vi "Eas_encryption.vi"(8 "error in":errorcluster, 10 "Key":string, 11 "User":string) -> (0 "Error out":errorcluster, 2 "Key":string, 3 "User":string)   [LabVIEW 2016]
uses:
  <vilib>/Alab Technologies/AES Crypto/Controls/Key Length.ctl
  <vilib>/Alab Technologies/AES Crypto/AES Crypto.lvlib
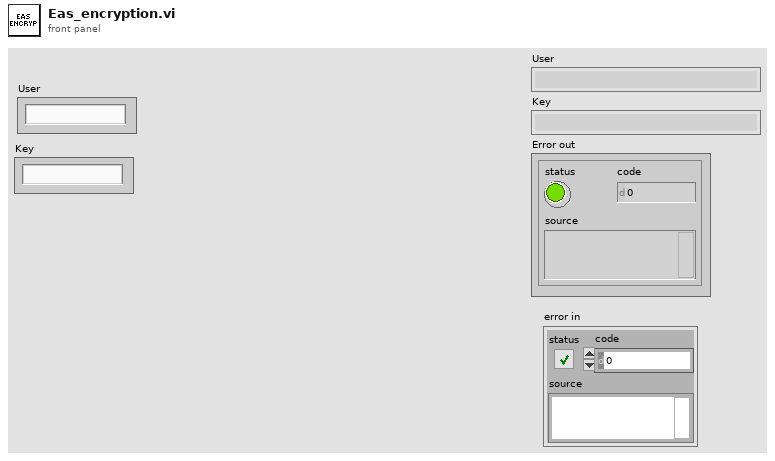
[diagram p1: front panel]
types:
  T1 = typedef "AES Crypto.lvlib/Key Length.ctl" = enum16{"128", "192", "256"}
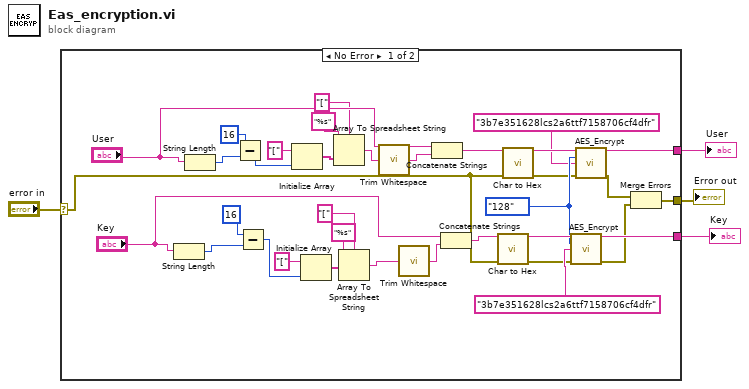
[diagram p0: block diagram]
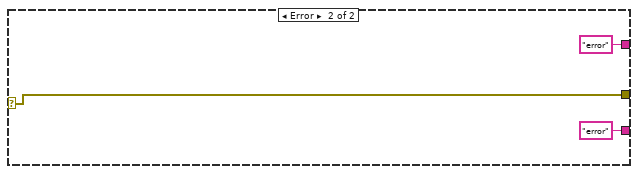
[diagram p2: hidden frame]
diagram:
  n1 = case shown="No Error" "error in" {
    selector: "error in" -> [w10 w42]
    tunnel: [w12 "error" ("Ciphertext (hex)")] -> w4
    tunnel: [w11 "error" ("Ciphertext (hex)")] -> w3
    tunnel: [w5 w42] -> w1
    frame No Error {
      w15 = Key_Length."128" ("Key length")
      n2 = String Length(string="Key") -> (length=w22:i32)
      n3 = String Length(string="User") -> (length=w24:i32)
      n4 = Subtract(x=16 ("y"), y=w24) -> (x-y=w36:i32)
      n5 = Subtract(x=16 ("y"), y=w22) -> (x-y=w38:i32)
      n6 = Initialize Array("[", w36) -> (w35:string[])
      n7 = Initialize Array("[", w38) -> (w34:string[])
      n8 = Array To Spreadsheet String(delimiter (Tab)="[", array=w35, 3:"%s" ("format string")) -> (spreadsheet string=w27:string)
      n9 = Array To Spreadsheet String(delimiter (Tab)="[", array=w34, 3:"%s" ("format string")) -> (spreadsheet string=w29:string)
      n10 = call <vilib>:"Trim Whitespace.vi"("string"=w27) -> ("trimmed string"=w26:string)  [unwired: 1 in]
      n11 = call <vilib>:"Trim Whitespace.vi"("string"=w29) -> ("trimmed string"=w28:string)  [unwired: 1 in]
      n12 = Concatenate Strings("User", w26) -> (w19:string)
      n13 = Concatenate Strings("Key", w28) -> (w17:string)
      n14 = call <vilib>:"Char to Hex.vi"("Input string (char)"=w17, "error in (no error)"=w10) -> ("Output string (hex)"=w16:string, "error out"=w9:errorcluster)  [unwired: 12 in]
      n15 = call <vilib>:"Char to Hex.vi"("Input string (char)"=w19, "error in (no error)"=w10) -> ("Output string (hex)"=w18:string, "error out"=w8:errorcluster)  [unwired: 12 in]
      n16 = call <vilib>:"AES_Encrypt.vi"("Plain text (hex)"=w16, "Key length"=w15, "Key (hex)"="3b7e351628lcs2a6ttf7158706cf4dfr", "Error In"=w9) -> ("Ciphertext (hex)"=w11:string, "Error out"=w7:errorcluster)  [unwired: 10 in]
      n17 = call <vilib>:"AES_Encrypt.vi"("Plain text (hex)"=w18, "Key length"=w15, "Key (hex)"="3b7e351628lcs2a6ttf7158706cf4dfr", "Error In"=w8) -> ("Ciphertext (hex)"=w12:string, "Error out"=w6:errorcluster)  [unwired: 10 in]
      n18 = Merge Errors(w6, w7) -> (w5:errorcluster)
    }
    frame Error {
    }
  }
  "User" <- w4
  "Key" <- w3
  "Error out" <- w1
